vi "Create KD Tree Float.vi"(5 "Overwrite Lib Path":path, 7 "flann_params":T1={"algorithm"=1, "checks"=32, "eps"=0.0, "sorted"=1, "max_neighbors"=-1, "cores"=0, "trees"=1, "leaf_max_size"=4, "branching"=32, "iterations"=5, "centers_init"=0, "cb_index"=0.5, "target_precision"=0.9, "build_weight"=0.01, "memory_weight"=0.0, "sample_fraction"=0.1, "table_number_"=12, "key_size_"=20, "multi_probe_level_"=2, "log_level"=0, "random_seed"=-1} {"algorithm" items=["FLANN_INDEX_LINEAR"=0, "FLANN_INDEX_KDTREE"=1, "FLANN_INDEX_KMEANS"=2, "FLANN_INDEX_COMPOSITE"=3, "FLANN_INDEX_KDTREE_SINGLE"=4, "FLANN_INDEX_HIERARCHICAL"=5, "FLANN_INDEX_LSH"=6, "FLANN_INDEX_SAVED"=254, "FLANN_INDEX_AUTOTUNED"=255]; "centers_init" items=["FLANN_CENTERS_RANDOM", "FLANN_CENTERS_GONZALES", "FLANN_CENTERS_KMEANSPP", "FLANN_CENTERS_GROUPWISE"]; "log_level" items=["FLANN_LOG_NONE", "FLANN_LOG_FATAL", "FLANN_LOG_ERROR", "FLANN_LOG_WARN", "FLANN_LOG_INFO", "FLANN_LOG_DEBUG"]}, 8 "error in (no error)":errorcluster, 11 "Points (Row-Vectors)":sgl[][](array[numeric])) -> (0 "error out":errorcluster, 3 "KD Tree Float out":refnum<class "KD Tree Float.lvclass">)   [LabVIEW 2020, in "KD Tree.lvlib" / "KD Tree Float.lvclass"]
uses:
  KD Tree Float.lvclass
  flann/Flann Params.ctl
  KD Tree.lvlib
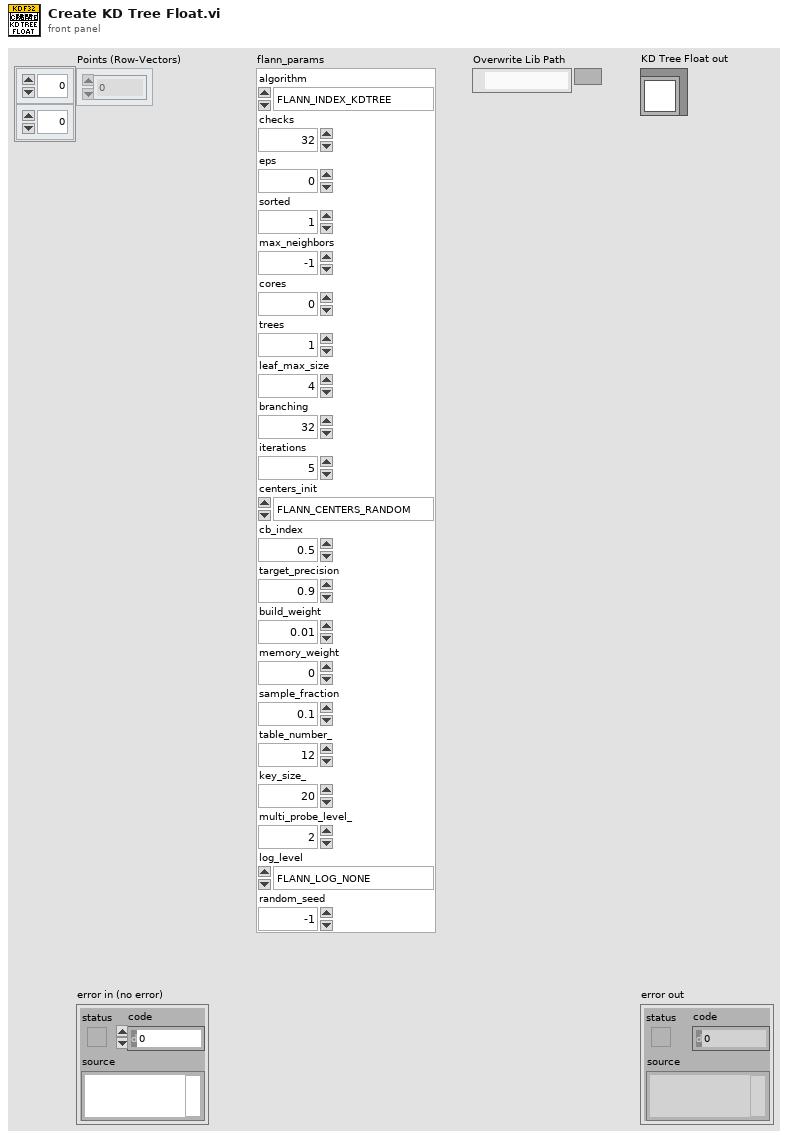
[diagram p1: front panel]
types:
  T1 = typedef "KD Tree.lvlib/Flann Params.ctl" = cluster{"algorithm":u32, "checks":i32, "eps":sgl, "sorted":i32, "max_neighbors":i32, "cores":i32, "trees":i32, "leaf_max_size":i32, "branching":i32, "iterations":i32, "centers_init":u32, "cb_index":sgl, "target_precision":sgl, "build_weight":sgl, "memory_weight":sgl, "sample_fraction":sgl, "table_number_":u32, "key_size_":u32, "multi_probe_level_":u32, "log_level":u32, "random_seed":i32}
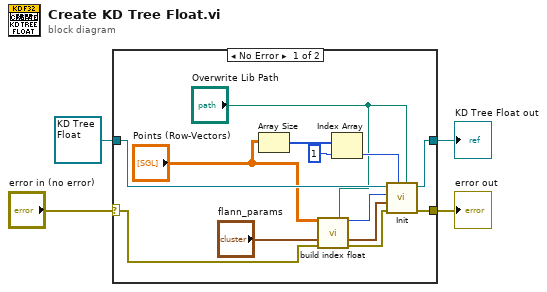
[diagram p0: block diagram]
diagram:
  n1 = case shown="No Error" "error in (no error)" {
    selector: "error in (no error)" -> [w17 w19]
    tunnel: [w15 w19] -> w1
    tunnel: [w13 w18] -> w3
    tunnel: refnum<class "KD Tree Float.lvclass"> refnum ("KD Tree Float in") -> [w14 w18]
    frame No Error {
      n2 = Array Size(array="Points (Row-Vectors)") -> (size(s)=w9:i32[])
      n3 = call "build index float.vi"("dataset"="Points (Row-Vectors)", "Overwrite Lib Path"="Overwrite Lib Path", "flann_params"="flann_params", "error in (no error)"=w17) -> ("Ref"=w12:u64, "flann_params"=w11:T1, "error out"=w16:errorcluster)  [unwired: 8 in, 1 out]
      n4 = Index Array(array=w9, index=1) -> (element=w6:i32)
      n5 = call-dynamic "Init.vi"("Overwrite Lib Path"="Overwrite Lib Path", "ndim"=w6, "error in (no error)"=w16, "flann_params"=w11, "index_ptr"=w12, "KD Tree in"=w14) -> ("error out"=w15:errorcluster, "KD Tree out"=w13:refnum<class "KD Tree Float.lvclass">)  [unwired: 4 in]
    }
    frame Error {
    }
  }
  "error out" <- w1
  "KD Tree Float out" <- w3
